vi "HB_SetLEDIntensity.vi"(0 "HBDevRef":T1, 9 "LED Intensity":u8=100, 11 "error in (no error)":errorcluster) -> (4 "HBDevRef":T1, 15 "error out":errorcluster)   [LabVIEW 2016]
uses:
  <vilib>/Rock Robotics/WPI/SerialPort/WPI_SerialPortRef.ctl
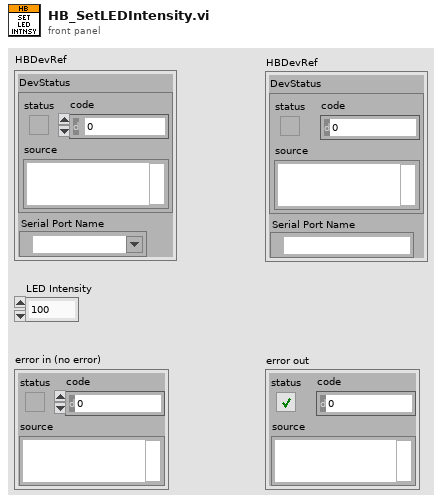
[diagram p1: front panel]
types:
  T1 = typedef "WPI_SerialPortRef.ctl" = cluster{"DevStatus":errorcluster, "Serial Port Name":refnum<visa-resource-name>}
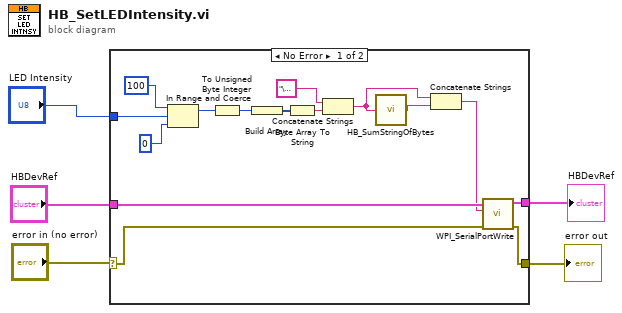
[diagram p0: block diagram]
diagram:
  n1 = case shown="No Error" "error in (no error)" {
    selector: "error in (no error)" -> [w6 w21]
    tunnel: "HBDevRef" -> [w20 w22]
    tunnel: [w19 w21] -> w4
    tunnel: [w18 w22] -> w3
    tunnel: "LED Intensity" -> [w11 _]
    frame No Error {
      n2 = In Range and Coerce(upper limit=100, x=w11, lower limit=0) -> (coerced(x)=w9:i32)  [unwired: 1 out]
      n3 = To Unsigned Byte Integer(number=w9) -> (unsigned 8bit integer=w17:u8)
      n4 = Build Array(w17) -> (w16:u8[])
      n5 = Byte Array To String(unsigned byte array=w16) -> (string=w13:string)
      n6 = Concatenate Strings("\u0016", w13) -> (w7:string)
      n7 = call <vilib>:"HB_SumStringOfBytes.vi"("String Of Bytes"=w7) -> ("Sum as String"=w8:string)
      n8 = Concatenate Strings(w7, w8) -> (w14:string)
      n9 = call <vilib>:"WPI_SerialPortWrite.vi"("error in (no error)"=w6, "Buffer"=w14, "SerialPortRef"=w20) -> ("error out"=w19:errorcluster, "SerialPortRef"=w18:T1)  [unwired: 6 in, 1 out]
    }
    frame Error {
    }
  }
  "error out" <- w4
  "HBDevRef" <- w3
